vi "IP配置.vi"() -> (2 "确定":bool)   [LabVIEW 2020]
uses:
  Global.vi
  <vilib>/Utility/file.llb/Write Delimited Spreadsheet (string).vi
panel:
  in  "Server(IP)":string="0"
  in  "取消":bool
  in  "确定":bool
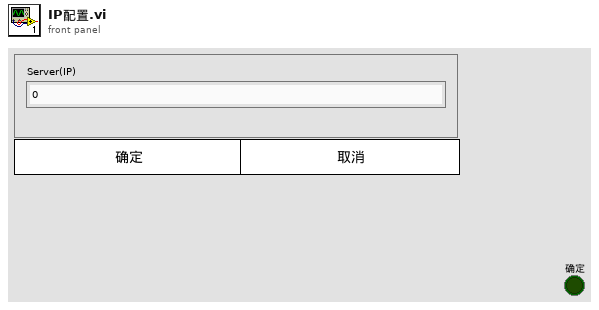
[diagram p1: front panel]
types:
  T1 = cluster{"Server":string, "audit_mode":string, "tsid":string, "model":string, "product":string, "test_station":string, "station_id":string, "test_station_name":string, "Webservice":string}
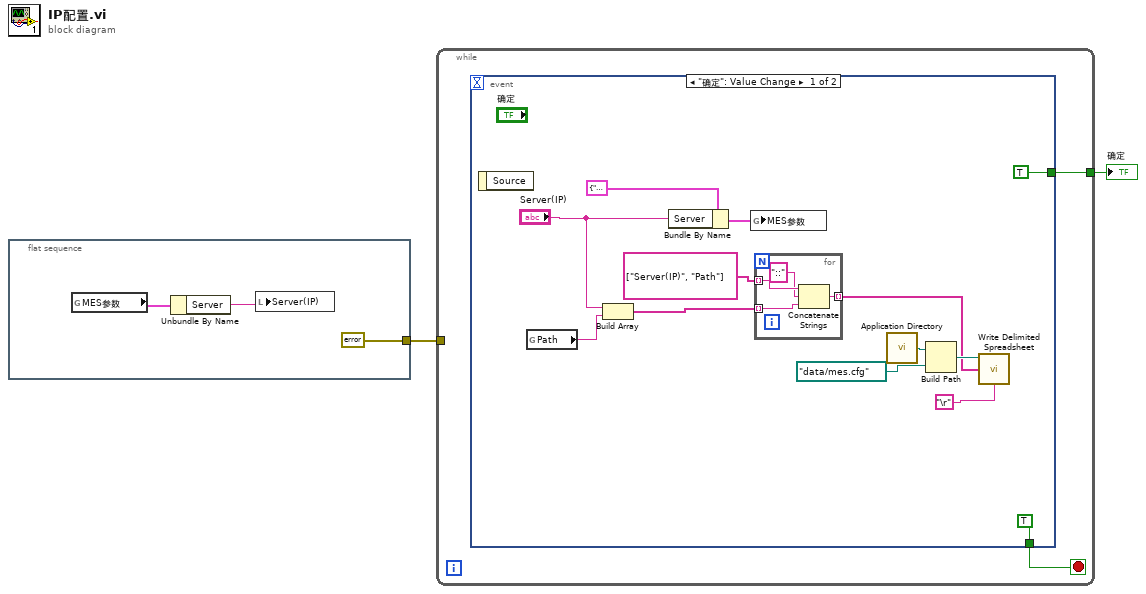
[diagram p0: block diagram]
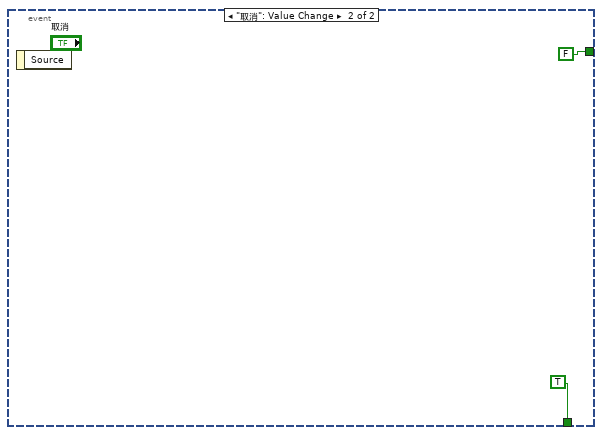
[diagram p2: hidden frame]
diagram:
  n1 = flat-sequence {
    tunnel: [errorcluster {"status"=FALSE, "code"=0, "source"=""} ("错误常量")] -> w1
    frame #0 {
      n2 = global read "Global.vi" "MES参数"() -> (w5:T1)
      n3 = Unbundle By Name(w5) -> ("Server"=w4:string)
      n4 = local write "Server(IP)"(w4) -> ()
    }
  }
  n5 = while {
    tunnel: [w6] -> w2
    tunnel: w1 -> [_]
    stop <- w7 stop-if-true
    n6 = event shown="[0] \"确定\": Value Change" {
      selector: _ -> [_ _]
      dyn-events: _ -> [_ _]
      timeout: _ -> [_ _]
      tunnel: [TRUE TRUE] -> w7
      tunnel: [TRUE FALSE] -> w6
      event "确定": Value Change {
        n7 = event-data() -> ()  [unwired: 1 in, 1 out]
        n8 = global read "Global.vi" "Path"() -> (w8:string)
        n9 = Build Array("Server(IP)", w8) -> (w11:string[])
        n10 = Bundle By Name(cluster=T1 {"Server"="http://10.32.13.198", "audit_mode"="0", "tsid"="3", "model"="4", "product"="5", "test_station"="6", "station_id"="7", "test_station_name"="8", "Webservice"="9"} ("MES参数"), "Server"="Server(IP)") -> (w17:T1)
        n11 = global write "Global.vi" "MES参数"(w17) -> ()
        n12 = for {
          tunnel: string[] ["Server(IP)", "Path"] ("转置的数组") -> [w24] mode=indexing
          tunnel: w11 -> [w22] mode=indexing
          tunnel: [w21] -> w10 mode=indexing
          n13 = Concatenate Strings(w24, "::" ("String"), w22) -> (w21:string)
        }
        n14 = call <vilib>:"Application Directory.vi"() -> ("Application Directory"=w14:path)
        n15 = Build Path(base path=w14, name or relative path=path "data/mes.cfg") -> (appended path=w13:path)
        n16 = call-poly <vilib>:"Write Delimited Spreadsheet.vi"("file path (dialog if empty)"=w13, "1D data"=w10, "delimiter (\\t)"="\r") -> ()  [unwired: 11 in, 2 out]
      }
      event "取消": Value Change {
        n17 = event-data() -> ()  [unwired: 1 in, 1 out]
      }
    }
  }
  "确定" <- w2
